vi "Absorb Give Up Checker.vi"(9 "Right Dist":dbl, 10 "Left Dist":dbl, 11 "Give Up Threshold":dbl) -> (3 "Give Up?":bool)   [LabVIEW 2014]
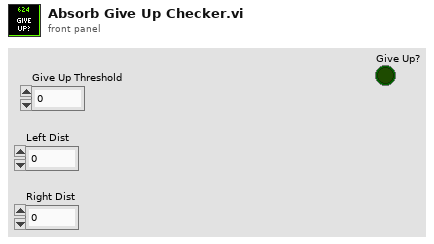
[diagram p1: front panel]
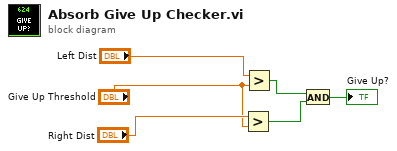
[diagram p0: block diagram]
diagram:
  n1 = Greater?(x="Right Dist", y="Give Up Threshold") -> (0:w2:bool)
  n2 = Greater?(x="Left Dist", y="Give Up Threshold") -> (0:w3:bool)
  n3 = And(x=w3, y=w2) -> (x .and. y?=→"Give Up?":bool)
